vi "_Get Interfaces.vi"(8 "error in (no error)":errorcluster, 11 "Baby in":refnum<class "Baby.lvclass">) -> (0 "error out":errorcluster, 2 "Concrete Interfaces":refnum<class "IUnknown.lvclass">[](array[class]), 3 "Baby out":refnum<class "Baby.lvclass">)   [LabVIEW 2009, in "Baby.lvclass"]
doc: "Returns an array of all the concrete interfaces implemented for the given interfaceable object. Child classes must override this vi."
uses:
  Baby.lvclass
  Source/IUnknown Class/IUnknown.lvclass
  ISleepableBaby/ISleepableBaby.lvclass
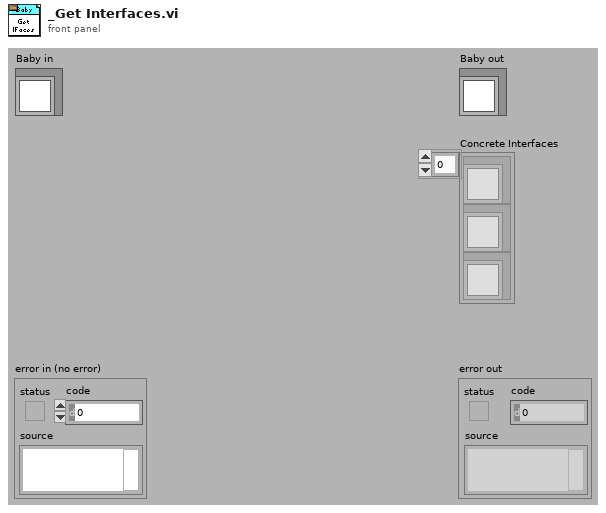
[diagram p1: front panel]
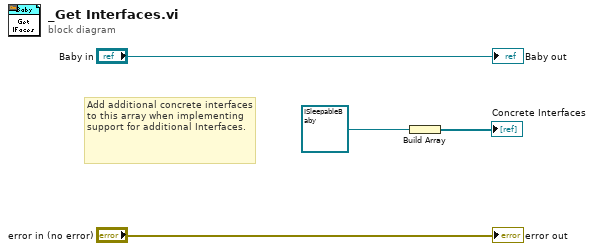
[diagram p0: block diagram]
diagram:
  # "Add additional concrete interfaces to this array when implementing support for additional Interfaces."
  n1 = Build Array(refnum<class "ISleepableBaby.lvclass"> refnum ("ISleepableBaby")) -> (→"Concrete Interfaces":refnum<class "ISleepableBaby.lvclass">[])
  "error out" <- "error in (no error)"
  "Baby out" <- "Baby in"
